vi "Get LV Classes.vi"(8 "error in (no error)":errorcluster, 11 "App reference":refnum<vi>) -> (0 "error out":errorcluster, 2 "LabVIEW Classes":refnum<vi>[](array[refnum]), 3 "dup App reference":refnum<vi>)   [LabVIEW 2009]
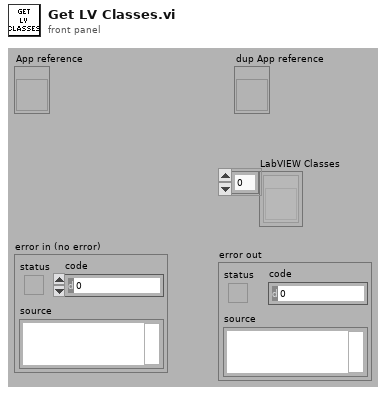
[diagram p1: front panel]
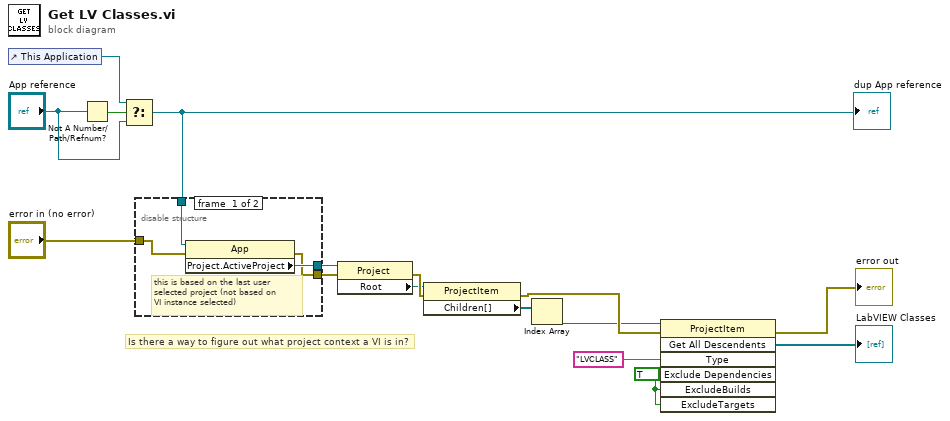
[diagram p0: block diagram]
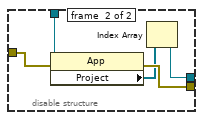
[diagram p2: hidden frame]
diagram:
  w10 = TRUE ("ExcludeDependencies")
  # "Is there a way to figure out what project context a VI is in?"
  n1 = control-ref of="This Application"() -> (w6:refnum<vi>)
  n2 = Not A Number/Path/Refnum?(number/path/refnum="App reference") -> (NaN/Path/Refnum?=w7:bool)
  n3 = Select(t=w6, s=w7, f="App reference") -> (s? t:f=w4:refnum<vi>)
  "dup App reference" <- w4
  n4 = disable-structure shown="Enabled" {
    disable-tunnel: w4 -> [w20 w25]
    disable-tunnel: "error in (no error)" -> [w19 w24]
    disable-tunnel: [w18 w21] -> w2
    disable-tunnel: [w17 w23] -> w1
    frame #0 {
      # "this is based on the last user\nselected project (not based on\nVI instance selected)"
      n5 = property class="App"(reference=w20, error in=w19) -> (error out=w17:errorcluster, "Project.ActiveProject"=w18:refnum<vi>)  [unwired: 1 out]
    }
    frame #1 {
      n6 = property class="App"(reference=w25, error in=w24) -> (error out=w23:errorcluster, "Project"=w22:refnum<vi>[])  [unwired: 1 out]
      n7 = Index Array(array=w22) -> (element=w21:refnum<vi>)  [unwired: 1 in]
    }
  }
  n8 = property class="Project"(reference=w2, error in=w1) -> (error out=w14:errorcluster, "Root"=w8:refnum<vi>)  [unwired: 1 out]
  n9 = property class="ProjectItem"(reference=w8, error in=w14) -> (error out=w15:errorcluster, "Children[]"=w11:refnum<vi>[])  [unwired: 1 out]
  n10 = Index Array(array=w11) -> (element=w12:refnum<vi>)  [unwired: 1 in]
  n11 = invoke class="ProjectItem" method="Get All Descendents"(reference=w12, error in=w15, "Type"="LVCLASS", "Exclude Dependencies"=w10, "ExcludeBuilds"=w10, "ExcludeTargets"=w10) -> (error out=→"error out":errorcluster, "All Descendents"=→"LabVIEW Classes":refnum<vi>[])  [unwired: 1 in, 5 out]
